vi "Validate Peripheral Channels.vi"(7 "Alias":string, 8 "error in (no error)":errorcluster, 9 "EVI (\"\")":string, 10 "Peripheral Name":string, 11 "FPGA Personality File Path":path) -> (0 "error out":errorcluster, 2 "Supported?":bool, 3 "Duplicated FPGA Personality File Path":path)   [LabVIEW 2021, in "Personality.lvlib"]
doc: "Checks if the channel of the peripheral/EVI is supported by the specified FPGA persoanlity file."
uses:
  <vilib>/myRIO/Common/FPGA Personality Framework/Personality.lvlib
  <vilib>/xml/Load XML File.vi
  <vilib>/xml/Close Reference(Node).vi
  <vilib>/xml/NI_XML.lvlib
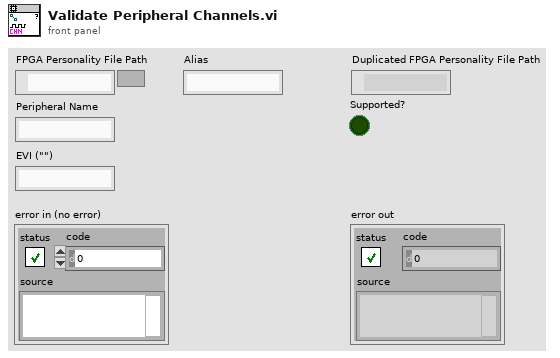
[diagram p1: front panel]
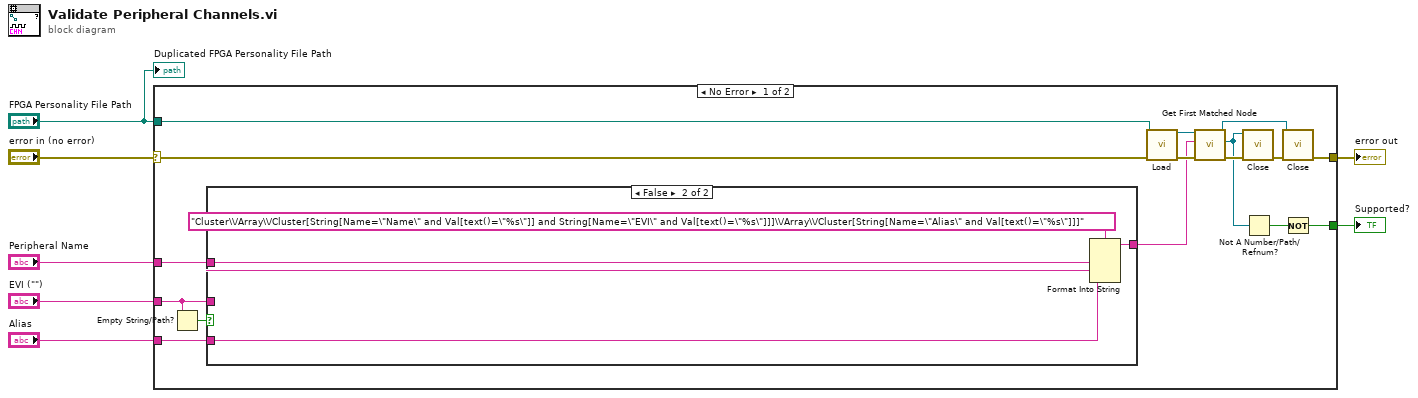
[diagram p0: block diagram]
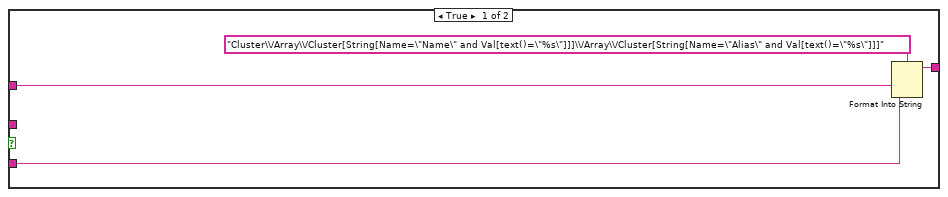
[diagram p2: hidden frame]
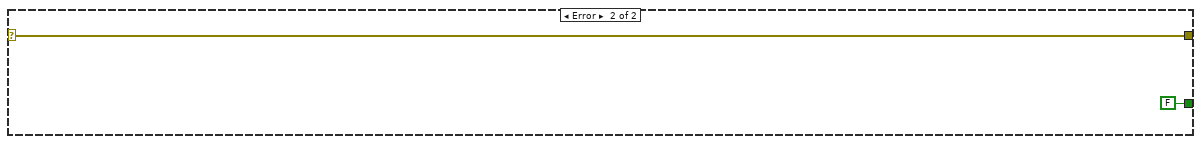
[diagram p3: hidden frame]
diagram:
  n1 = case shown="No Error" "error in (no error)" {
    selector: "error in (no error)" -> [w23 w34]
    tunnel: [w22 w34] -> w6
    tunnel: "FPGA Personality File Path" -> [w21 _]
    tunnel: "Peripheral Name" -> [w20 _]
    tunnel: "Alias" -> [w19 _]
    tunnel: [w18 FALSE] -> w2
    tunnel: "EVI (\"\")" -> [w8 _]
    frame No Error {
      n2 = Empty String/Path?(string/path=w8) -> (empty?=w9:bool)
      n3 = case shown="False" w9 {
        tunnel: w20 -> [w27 w32]
        tunnel: w19 -> [w26 w29]
        tunnel: [w25 w31] -> w15
        tunnel: w8 -> [_ w28]
        frame True {
          n4 = Format Into String(format string="Cluster\\/Array\\/Cluster[String[Name=\"Name\" and Val[text()=\"%s\"]]]\\/Array\\/Cluster[String[Name=\"Alias\" and Val[text()=\"%s\"]]]", w27, w26) -> (resulting string=w25:string)  [unwired: 2 in, 1 out]
        }
        frame False {
          n5 = Format Into String(format string="Cluster\\/Array\\/Cluster[String[Name=\"Name\" and Val[text()=\"%s\"]] and String[Name=\"EVI\" and Val[text()=\"%s\"]]]\\/Array\\/Cluster[String[Name=\"Alias\" and Val[text()=\"%s\"]]]", w32, w28, w29) -> (resulting string=w31:string)  [unwired: 2 in, 1 out]
        }
      }
      n6 = call-poly <vilib>:"Load.vi"("path to XML document"=w21, "error in (no error)"=w23) -> ("DOM document out"=w17:refnum<k20>, "error out"=w16:errorcluster)  [unwired: 11 in, 1 out]
      n7 = call <vilib>:"Get First Matched Node.vi"("error in (no error)"=w16, "XPath expression"=w15, "node in"=w17) -> ("error out"=w13:errorcluster, "node result"=w11:refnum<k20>, "node out"=w12:refnum<k20>)  [unwired: 6 in]
      n8 = call-poly <vilib>:"Close.vi"("error in (no error)"=w13, "node"=w11) -> ("error out"=w14:errorcluster)  [unwired: 7 in]
      n9 = Not A Number/Path/Refnum?(number/path/refnum=w11) -> (NaN/Path/Refnum?=w10:bool)
      n10 = call-poly <vilib>:"Close.vi"("error in (no error)"=w14, "node"=w12) -> ("error out"=w22:errorcluster)  [unwired: 7 in]
      n11 = Not(x=w10) -> (.not. x?=w18:bool)
    }
    frame Error {
    }
  }
  "error out" <- w6
  "Supported?" <- w2
  "Duplicated FPGA Personality File Path" <- "FPGA Personality File Path"
